vi "XML to Debugging.vi"(0 "XML Data":string) -> ()   [LabVIEW 2013]
uses:
  Types/Debugging.ctl
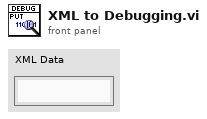
[diagram p1: front panel]
types:
  T1 = typedef "Debugging.ctl" = cluster{"In Place Debug Enabled":bool, "Version":string}
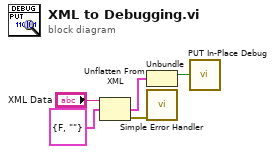
[diagram p0: block diagram]
diagram:
  n1 = Unflatten From XML(xml string="XML Data", type=T1 {"In Place Debug Enabled"=FALSE, "Version"=""} ("Debugging")) -> (value=w2:T1, error out=w5:errorcluster)  [unwired: 1 in]
  n2 = Unbundle(w2) -> ("In Place Debug Enabled"=w1:bool)  [unwired: 1 out]
  n3 = call <vilib>:"Simple Error Handler.vi"("error in (no error)"=w5) -> ()  [unwired: 4 in, 5 out]
  n4 = call "PUT In-Place Debug.vi"("In Place Debug Enabled"=w1) -> ()
